vi "setSysTopics.vi"(8 "error in (no error)":errorcluster, 11 "MQTTclient in":refnum<class "MQTTclient.lvclass">) -> (0 "error out":errorcluster, 2 "List of topics":string, 3 "MQTTclient out":refnum<class "MQTTclient.lvclass">)   [LabVIEW 2017, in "MQTTclient.lvclass"]
uses:
  MQTTclient.lvclass
  MQTTclient.lvclass/MQTTclient.ctl
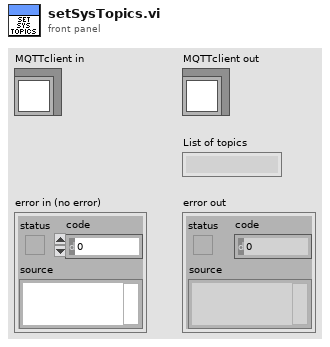
[diagram p1: front panel]
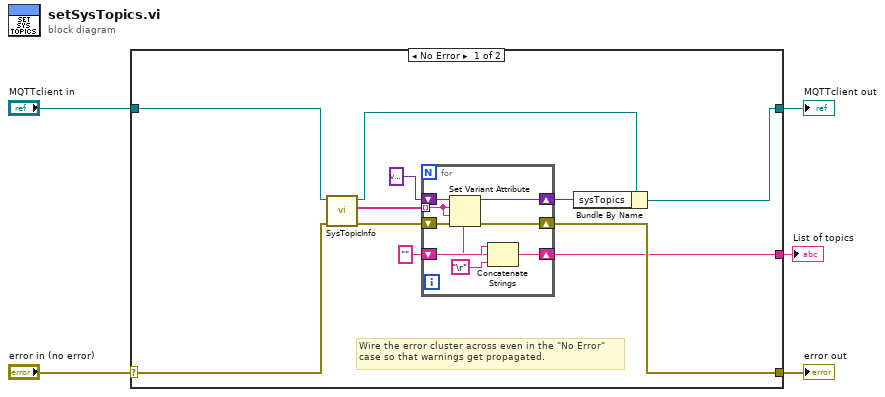
[diagram p0: block diagram]
diagram:
  n1 = case shown="No Error" "error in (no error)" {
    selector: "error in (no error)" -> [w8 w26]
    tunnel: [w9 w26] -> w4
    tunnel: [w10 w25] -> w2
    tunnel: "MQTTclient in" -> [w13 w25]
    tunnel: [w6 _] -> w1
    frame No Error {
      # "Wire the error cluster across even in the \"No Error\"\ncase so that warnings get propagated."
      n2 = call-dynamic "SysTopicInfo.vi"("error in (no error)"=w8, "MQTTclient in"=w13) -> ("error out"=w16:errorcluster, "Sys Topics"=w14:string[], "MQTTclient out"=w12:refnum<class "MQTTclient.lvclass">)  [unwired: 6 in, 1 out]
      n3 = for {
        tunnel: w14 -> [w17] mode=indexing
        shift-right: [w22] -> w11
        shift-left: variant -> [w24]
        shift-right: [w21] -> w9
        shift-left: w16 -> [w23]
        shift-right: [w19] -> w6
        shift-left: "" -> [w20]
        n4 = Set Variant Attribute(Variant=w24, name=w17, value=w17, error in=w23) -> (Variant out=w22:variant, error out=w21:errorcluster)  [unwired: 1 out]
        n5 = Concatenate Strings(w20, w17, "\r") -> (w19:string)
      }
      n6 = Bundle By Name(cluster=w12, "sysTopics"=w11) -> (w10:refnum<class "MQTTclient.lvclass">)
    }
    frame Error {
    }
  }
  "error out" <- w4
  "MQTTclient out" <- w2
  "List of topics" <- w1
